vi "Tester.vi"() -> ()   [LabVIEW 2014]
uses:
  <vilib>/Utility/file.llb/Read From Spreadsheet File (DBL).vi
panel:
  out "W":dbl[][](array[numeric])
  out "A":dbl[][](array[numeric])
  in  "Data File":path
  in  "Variables":T1={"s_verbose"=enum."On", "displayInterval"=1.0, "displayMode"=enum."On", "sampleSize"=1.0, "guess"=[[1.0]], "initState"=enum."rand", "maxFinetune"=100.0, "maxNumIteration"=100.0, "epsilon"=0.0001, "stabilization"=enum."On", "myy"=1.0, "a1"=1.0, "a2"=1.0, "finetune"=enum."pow3", "g"=enum."pow3", "approach"=enum."delf"}
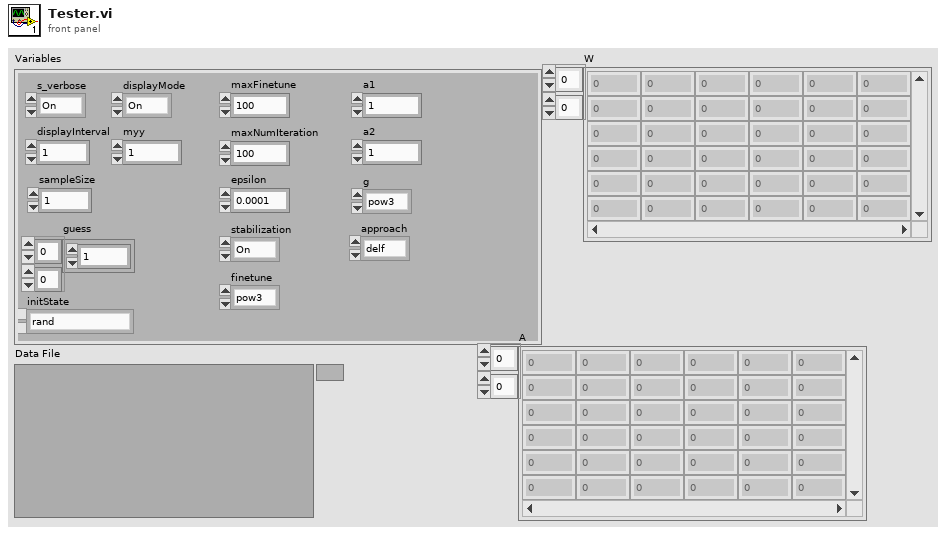
[diagram p1: front panel]
types:
  T1 = cluster{"s_verbose":enum16{"Off", "On"}, "displayInterval":dbl, "displayMode":enum16{"Off", "On"}, "sampleSize":dbl, "guess":dbl[][], "initState":enum16{"rand", "guess"}, "maxFinetune":dbl, "maxNumIteration":dbl, "epsilon":dbl, "stabilization":enum16{"Off", "On"}, "myy":dbl, "a1":dbl, "a2":dbl, "finetune":enum16{"pow3", "tanh", "gauss", "skew", "off"}, "g":enum16{"pow3", "tanh", "gauss", "skew"}, "approach":enum16{"symm", "delf"}}
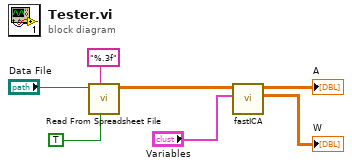
[diagram p0: block diagram]
diagram:
  n1 = call-poly <vilib>:"Read From Spreadsheet File.vi"("transpose (no:F)"=TRUE, "format (%.3f)"="%.3f", "file path (dialog if empty)"="Data File") -> ("all rows"=w6:dbl[][])  [unwired: 4 in, 4 out]
  n2 = call "fastICA.vi"("Variables"="Variables", "Input Data (X)"=w6) -> ("W"=→"W":dbl[][], "A"=→"A":dbl[][])  [unwired: 8 in]
